vi "Save Project.vi"(0 "Project reference":refnum<vi>, 5 "MeasurementCore reference":refnum<vi>, 7 "Project path":path, 11 "error in (no error)":errorcluster) -> (15 "error out":errorcluster)   [LabVIEW 2021]
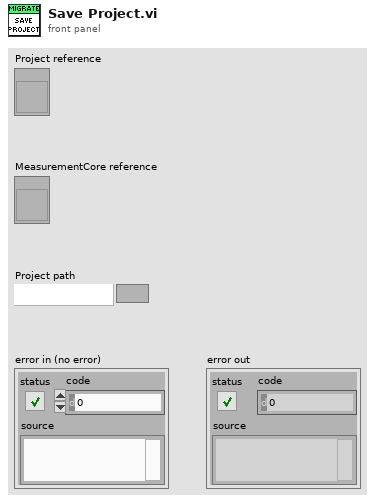
[diagram p1: front panel]
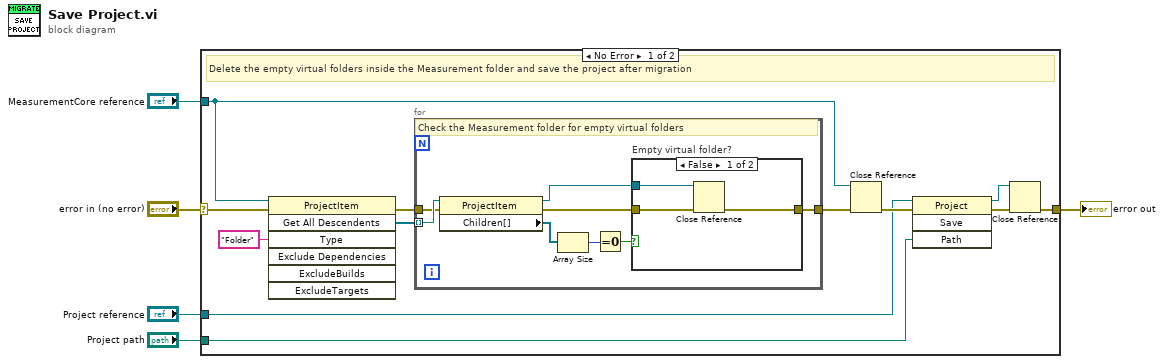
[diagram p0: block diagram]
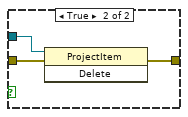
[diagram p2: hidden frame]
diagram:
  n1 = case shown="No Error" "error in (no error)" {
    selector: "error in (no error)" -> [w14 w32]
    tunnel: [w16 w32] -> w5
    tunnel: "Project path" -> [w8 _]
    tunnel: "MeasurementCore reference" -> [w9 _]
    tunnel: "Project reference" -> [w6 _]
    frame No Error {
      # "Delete the empty virtual folders inside the Measurement folder and save the project after migration"
      n2 = invoke class="ProjectItem" method="Get All Descendents"(reference=w9, error in=w14, "Type"="Folder") -> (error out=w11:errorcluster, "All Descendents"=w12:refnum<vi>[])  [unwired: 4 in, 5 out]
      n3 = for {
        tunnel: w12 -> [w25] mode=indexing
        tunnel: w11 -> [w24]
        tunnel: [w18] -> w10
        # "Check the Measurement folder for empty virtual folders"
        n4 = property class="ProjectItem"(reference=w25, error in=w24) -> (reference out=w19:refnum<vi>, error out=w21:errorcluster, "Children[]"=w23:refnum<vi>[])
        n5 = Array Size(array=w23) -> (size(s)=w22:i32)
        n6 = Equal To 0?(x=w22) -> (x = 0?=w20:bool)
        n7 = case "Empty virtual folder?" shown="False" w20 {
          tunnel: w21 -> [w28 w31]
          tunnel: w19 -> [w27 w30]
          tunnel: [w26 w29] -> w18
          frame False {
            n8 = Close Reference(reference=w27, error in (no error)=w28) -> (error out=w26:errorcluster)
          }
          frame True {
            n9 = invoke class="ProjectItem" method="Delete"(reference=w30, error in=w31) -> (error out=w29:errorcluster)  [unwired: 1 in, 2 out]
          }
        }
      }
      n10 = Close Reference(reference=w9, error in (no error)=w10) -> (error out=w7:errorcluster)
      n11 = invoke class="Project" method="Save"(reference=w6, error in=w7, "Path"=w8) -> (reference out=w17:refnum<vi>, error out=w15:errorcluster)  [unwired: 1 in, 2 out]
      n12 = Close Reference(reference=w17, error in (no error)=w15) -> (error out=w16:errorcluster)
    }
    frame Error {
    }
  }
  "error out" <- w5
